vi "Collection (Array).vi"(8 "error in (no error)":errorcluster, 10 "Array":refnum<class "Readable.lvclass">[](array[class]), 11 "Collection.lvclass in":refnum<class "Collection.lvclass">) -> (0 "error out":errorcluster, 3 "Collection.lvclass out":refnum<class "Collection.lvclass">)   [LabVIEW 2009, in "Collection.lvclass"]
uses:
  Collection.lvclass
  Readable/Readable.lvclass
  Collection.lvclass/Collection.ctl
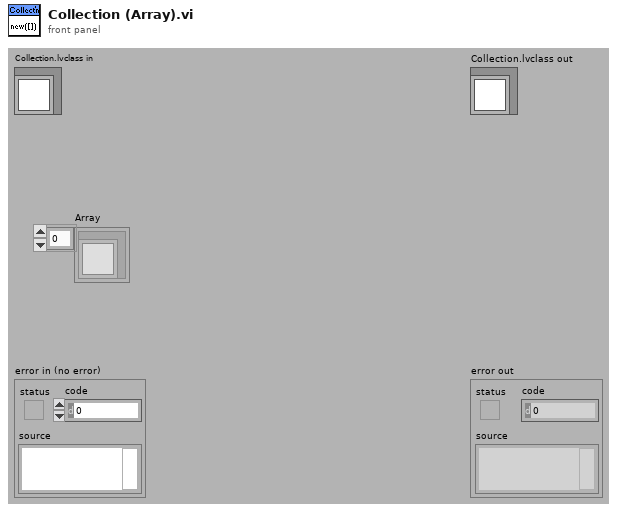
[diagram p1: front panel]
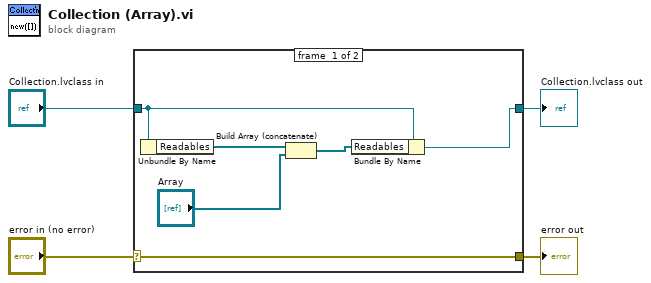
[diagram p0: block diagram]
diagram:
  n1 = case shown="No Error" "error in (no error)" {
    selector: "error in (no error)" -> [w10 w11]
    tunnel: [w10 w11] -> w3
    tunnel: [w9 w12] -> w1
    tunnel: "Collection.lvclass in" -> [w8 w12]
    frame #0 {
      n2 = Unbundle By Name(w8) -> ("Readables"=w6:refnum<class "Readable.lvclass">[])
      n3 = Build Array (concatenate)(w6, "Array") -> (w5:refnum<class "Readable.lvclass">[])
      n4 = Bundle By Name(cluster=w8, "Readables"=w5) -> (w9:refnum<class "Collection.lvclass">)
    }
    frame #1 {
    }
  }
  "error out" <- w3
  "Collection.lvclass out" <- w1
